vi "两数之和.vi"() -> ()   [LabVIEW 2020]
panel:
  in  "target 3":dbl
  in  "target 2":dbl
  in  "target":dbl
  in  "x3":dbl
  in  "x2":dbl
  in  "x1":dbl
  out "result":bool=TRUE
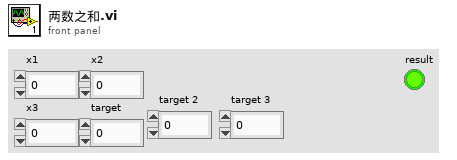
[diagram p1: front panel]
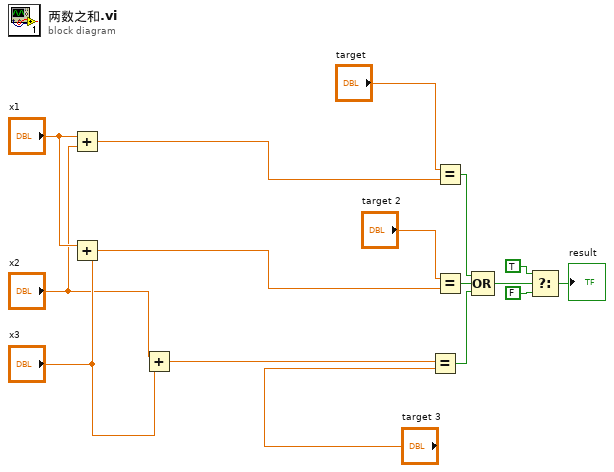
[diagram p0: block diagram]
diagram:
  n1 = Add(x="x1", y="x2") -> (x+y=w12:dbl)
  n2 = Add(x="x1", y="x3") -> (x+y=w6:dbl)
  n3 = Add(x="x2", y="x3") -> (x+y=w4:dbl)
  n4 = Equal?(x=w4, y="target 3") -> (x = y?=w3:bool)
  n5 = Equal?(x="target", y=w12) -> (x = y?=w11:bool)
  n6 = Equal?(x="target 2", y=w6) -> (x = y?=w5:bool)
  n7 = Compound Arithmetic op=OR ("复合运算")(w11, w5, w3) -> (w2:bool)
  n8 = Select(t=TRUE, s=w2, f=FALSE) -> (s? t:f=→"result":bool)
